vi "音高列表.vi"() -> ()   [LabVIEW 2015]
panel:
  out "size(s)":i32
  out "Array":dbl[](array[numeric])
  out "frequence":dbl
  in  "MIDI":ext format="%#_13g"
  out "MIDI":dbl
  in  "frequence":ext format="%#_13g"
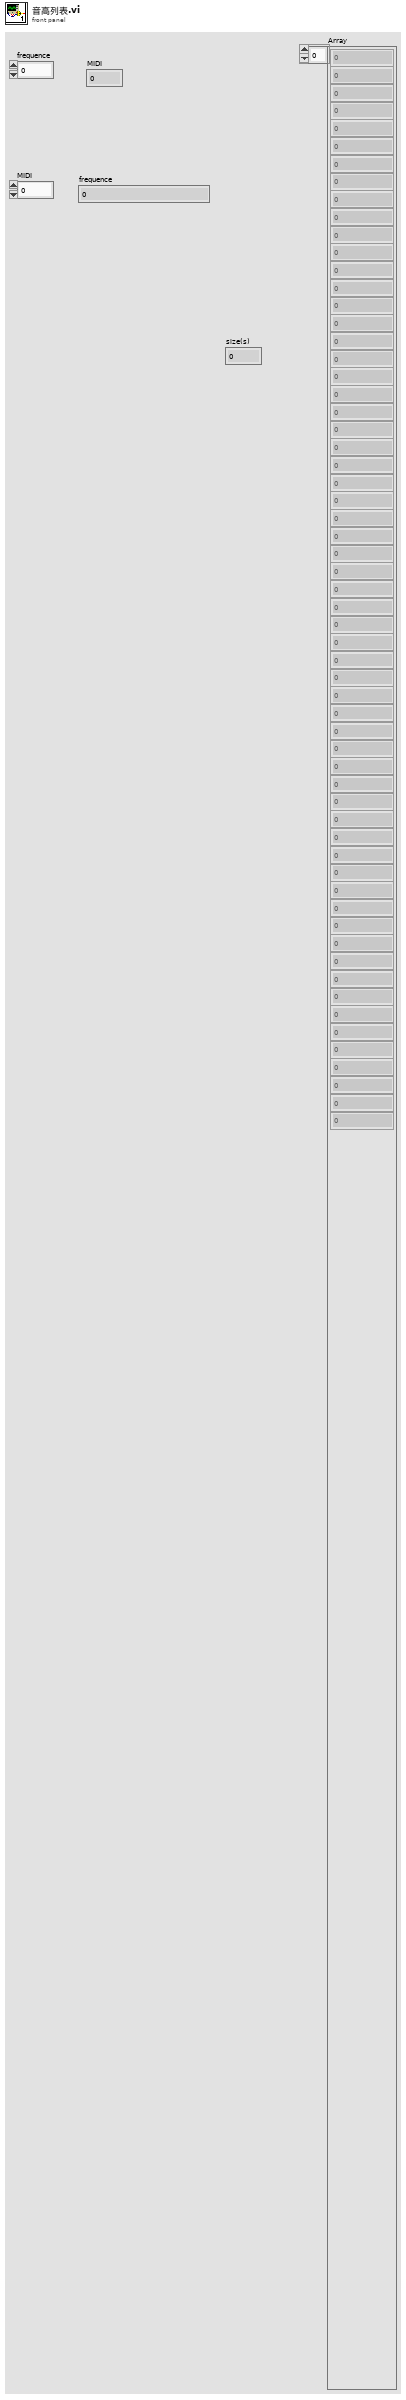
[diagram p1: front panel]
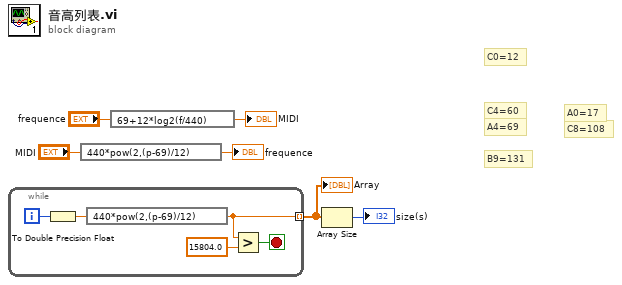
[diagram p0: block diagram]
diagram:
  # "C8=108"
  # "A0=17"
  # "B9=131"
  # "C4=60"
  # "C0=12"
  # "A4=69"
  n1 = while {
    tunnel: [w9] -> w5 mode=indexing
    i -> [w8]
    stop <- w10 stop-if-true
    n2 = To Double Precision Float(number=w8) -> (double precision float=w7:dbl)
    n3 = expression code="440*pow(2,(p-69)/12)"(w7) -> (w9:dbl)
    n4 = Greater?(x=w9, y=15804.0) -> (0:w10:bool)
  }
  "Array" <- w5
  n5 = expression code="440*pow(2,(p-69)/12)"("MIDI") -> (→"frequence":ext)
  n6 = expression code="69+12*log2(f/440)"("frequence") -> (→"MIDI":ext)
  n7 = Array Size(array=w5) -> (size(s)=→"size(s)":i32)
